vi "main2.vi"() -> ()   [LabVIEW 2014]
uses:
  src/user.lib/_NEVSTOP/GlobalStop/_gStop.vi
  src/user.lib/_NEVSTOP/GlobalStop/GSTOP.lvlib
panel:
  in  "stop 1 IN Main Loop":bool
  in  "stop all":bool
  out "loop main":i32
  in  "stop 2":bool
  out "loop status":i32
  out "loop2":i32
  out "loop1":i32
  in  "stop 1":bool
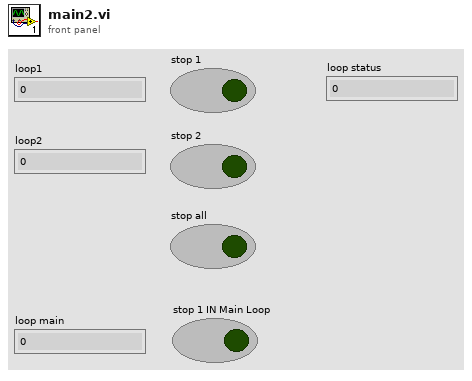
[diagram p1: front panel]
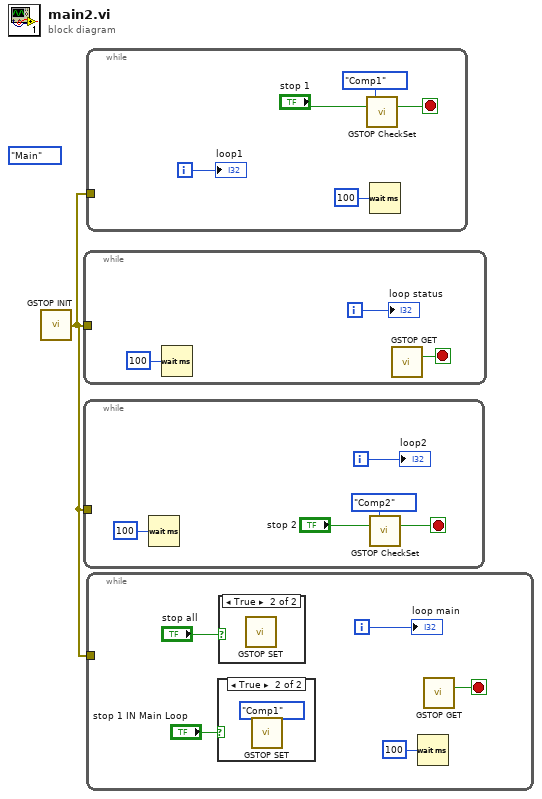
[diagram p0: block diagram]
diagram:
  (unwired) enum16{"Main", "Comp1", "Comp2"}."Main"
  n1 = call "GSTOP INIT.vi"() -> ("error out"=w1:errorcluster)  [unwired: 15 in]
  n2 = while {
    tunnel: w1 -> [_]
    i -> [w2]
    stop <- w3 stop-if-true
    n3 = Wait (ms)(milliseconds to wait=100) -> ()  [unwired: 1 out]
    n4 = call "GSTOP GET.vi"() -> ("stop"=w3:bool)  [unwired: 14 in, 1 out]
    "loop status" <- w2
  }
  n5 = while {
    tunnel: w1 -> [_]
    i -> [w6]
    stop <- w8 stop-if-true
    n6 = Wait (ms)(milliseconds to wait=100) -> ()  [unwired: 1 out]
    n7 = call "GSTOP CheckSet.vi"("index(-1 for All)"=enum16{"Main", "Comp1", "Comp2"}."Comp2", "stop value"="stop 2") -> ("stop"=w8:bool)  [unwired: 12 in, 1 out]
    "loop2" <- w6
  }
  n8 = while {
    tunnel: w1 -> [_]
    i -> [w14]
    stop <- w12 stop-if-true
    n9 = call "GSTOP CheckSet.vi"("index(-1 for All)"=enum16{"Main", "Comp1", "Comp2"}."Comp1", "stop value"="stop 1") -> ("stop"=w12:bool)  [unwired: 12 in, 1 out]
    n10 = Wait (ms)(milliseconds to wait=100) -> ()  [unwired: 1 out]
    "loop1" <- w14
  }
  n11 = while {
    tunnel: w1 -> [_]
    i -> [w19]
    stop <- w16 stop-if-true
    n12 = case shown="True" "stop 1 IN Main Loop" {
      frame False {
      }
      frame True {
        n13 = call "GSTOP SET.vi"("index(-1 for All)"=enum16{"Main", "Comp1", "Comp2"}."Comp1") -> ()  [unwired: 14 in, 1 out]
      }
    }
    n14 = case shown="True" "stop all" {
      frame False {
      }
      frame True {
        n15 = call "GSTOP SET.vi"() -> ()  [unwired: 15 in, 1 out]
      }
    }
    n16 = Wait (ms)(milliseconds to wait=100) -> ()  [unwired: 1 out]
    n17 = call "GSTOP GET.vi"() -> ("stop"=w16:bool)  [unwired: 14 in, 1 out]
    "loop main" <- w19
  }
